vi "Packet_generator.vi"(0 "user  bitstream":i8[](array[numeric])=[1], 1 "Samples pr burst":i32, 2 "Bits per sample":i32, 3 "Message Bits":i32) -> (7 "Array":i8[][](array[numeric]))   [LabVIEW 2014]
uses:
  <vilib>/addons/Modulation/Digital/General/MT Generate Bits (Galois, PN Order).vi
  <vilib>/addons/Modulation/Digital/Support/Common/Validators/mod_Generate Bits Validate.vi
  <vilib>/addons/Modulation/Analog/support/mod_Set Error Source.vi
  <vilib>/addons/Modulation/Digital/General/subVIs/mod_Generate Bits PN Sequence.vi
  <vilib>/addons/Modulation/niDMT.lvlib
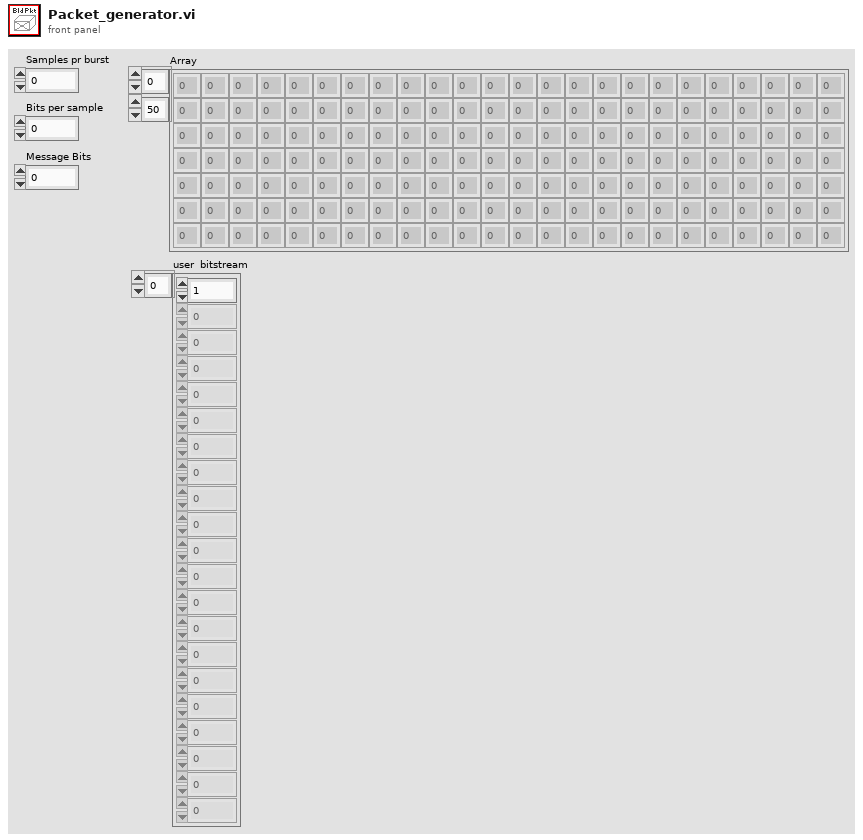
[diagram p1: front panel]
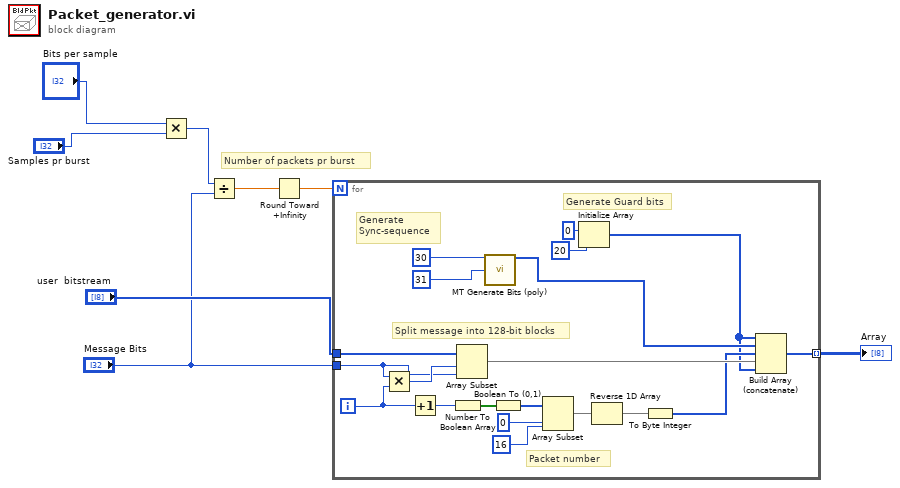
[diagram p0: block diagram]
diagram:
  # "Number of packets pr burst"
  n1 = Multiply(x="Bits per sample", y="Samples pr burst") -> (x*y=w1:i32)
  n2 = Divide(x=w1, y="Message Bits") -> (x/y=w5:dbl)
  n3 = Round Toward +Infinity(x=w5) -> (ceil(x): smallest int >= x=w4:dbl)
  n4 = for {
    N: w4 -> [_]
    tunnel: "Message Bits" -> [w22]
    tunnel: "user  bitstream" -> [w23]
    tunnel: [w28] -> w7 mode=indexing
    i -> [w14]
    # "Split message into 128-bit blocks"
    # "Packet number"
    # "Generate Guard bits"
    # "Generate\nSync-sequence"
    n5 = Multiply(x=w22, y=w14) -> (x*y=w24:i32)
    n6 = Increment(x=w14) -> (x+1=w25:i32)
    n7 = Number To Boolean Array(number=w25) -> (Boolean array=w26:bool[])
    n8 = Array Subset(array=w23, index=w24, length=w22) -> (w21:i8[])
    n9 = call-poly <vilib>:"MT Generate Bits (poly).vi"("total bits (128)"=30, "PN sequence order (9)"=31) -> ("output bit stream"=w19:i8[])  [unwired: 11 in, 2 out]
    n10 = Boolean To (0,1)(Boolean=w26) -> (0, 1=w13:i16[])
    n11 = Array Subset(array=w13, index=0, length=16) -> (w10:i16[])
    n12 = Initialize Array(0 ("Numeric"), 20 ("dimension size")) -> (w16:i32[])
    n13 = Reverse 1D Array(array=w10) -> (reversed array=w9:i16[])
    n14 = To Byte Integer(number=w9) -> (8bit integer=w20:i8[])
    n15 = Build Array (concatenate)(w16, w19, w20, w21, w16) -> (w28:i32[])
  }
  "Array" <- w7
